vi "GetDisplayForRect.vi"(8 "No Error":errorcluster, 11 "Rect":T1) -> (0 "Error Out":errorcluster, 3 "DisplayID":T2)   [LabVIEW 2024, in "SDL3.lvlib" / "Video.lvlib"]
doc: "<B>Summary</B>\nGet the display primarily containing a rect."
uses:
  Video.lvlib
  Lib/SDL3-32.dll
  Error/Error.lvlib
  DisplayID--integer.ctl
  Rect/Rect--cluster.ctl
  Rect/Rect.lvlib
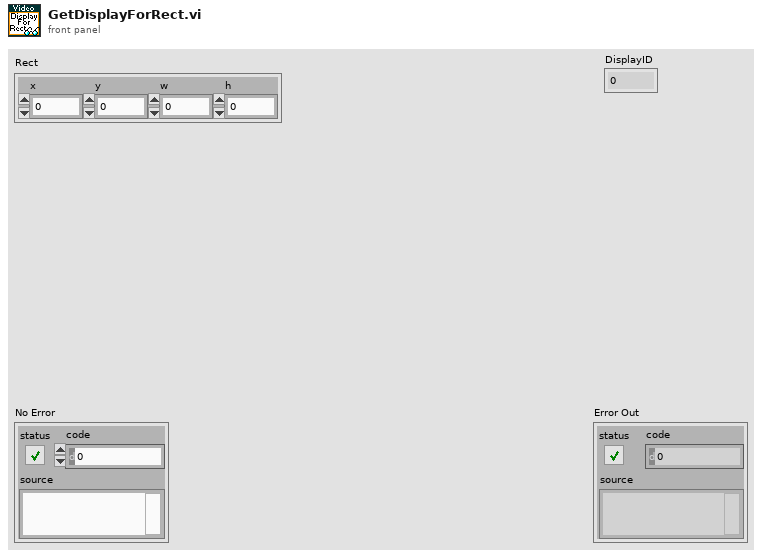
[diagram p1: front panel]
types:
  T1 = typedef "SDL3.lvlib/Rect.lvlib/Rect--cluster.ctl" = cluster{"x":i32, "y":i32, "w":i32, "h":i32}
  T2 = typedef "SDL3.lvlib/Video.lvlib/DisplayID--integer.ctl" = u32
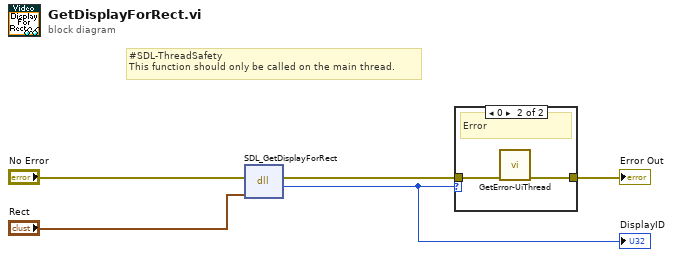
[diagram p0: block diagram]
diagram:
  # "#SDL-ThreadSafety\nThis function should only be called on the main thread."
  n1 = dll-call lib="C:/Users/Thomas/Documents/Projects/LV-SDL3/Lib/SDL3-*.*" fn="SDL_GetDisplayForRect"(error in="No Error", "rect"="Rect") -> (error out=w3:errorcluster, "return type"=w2:u32)  [unwired: 3 in, 1 out]
  "DisplayID" <- w2
  n2 = case shown="0" w2 {
    tunnel: w3 -> [w6 w8]
    tunnel: [w6 w7] -> w4
    frame Default {
      # "Ok"
    }
    frame 0 {
      # "Error"
      n3 = call "GetError-UiThread.vi"("No Error"=w8) -> ("error out"=w7:errorcluster)  [unwired: 10 in]
    }
  }
  "Error Out" <- w4
